vi "Test SendLogRecordsMakesThemAvailableInLoki.vi"(8 "error in (no error)":errorcluster) -> (0 "error out":errorcluster)   [LabVIEW 2017, in "UT_LokiHandler.lvlib"]
doc: "Template for an unit test with caraya in the \"Given, When, Then\" structure from James."
uses:
  UT_LokiHandler.lvlib
  Source/HSE-Logger/LogRecord/LogRecord.lvclass/LogRecord.ctl
  <vilib>/ErrorRing/Error Ring.xnode
  Source/HSE-Logger/Handler/LokiHandler/LokiHandler.lvclass
  <vilib>/addons/_JKI Toolkits/Caraya/classes/Test/Test.lvclass
  <vilib>/addons/_JKI Toolkits/Caraya/classes/Assert/Assert.lvclass
  Source/HSE-Logger/LogRecord/LogRecord.lvclass
  Source/HSE-Logger/LogLevel.ctl
  Source/HSE-Logger/hse-logger.lvlib
  <vilib>/Utility/error.llb/Error Cluster From Error Code.vi
  Source/HSE-Logger/Formatter/LokiJsonFormatter/LokiJsonFormatter.lvclass
  <vilib>/httpClient/LabVIEWHTTPClient.lvlib
  <vilib>/addons/_JKI Toolkits/Caraya/classes/Assert/Assert Greater_Variant.vi
  <vilib>/httpClient/POSTBuffer.vi
panel:
  # "Connector Pane"
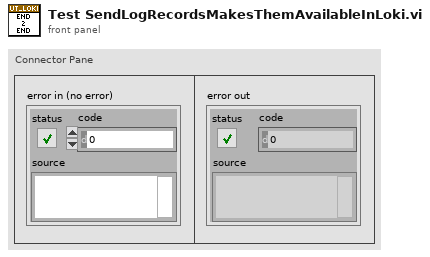
[diagram p1: front panel]
types:
  T1 = typedef "hse-logger.lvlib/LogLevel.ctl" = enum16{"DEBUG", "INFO", "WARNING", "ERROR", "CRITICAL"}
  T2 = typedef "LabVIEWHTTPClient.lvlib/ClientHandle.ctl" = refnum<k1>
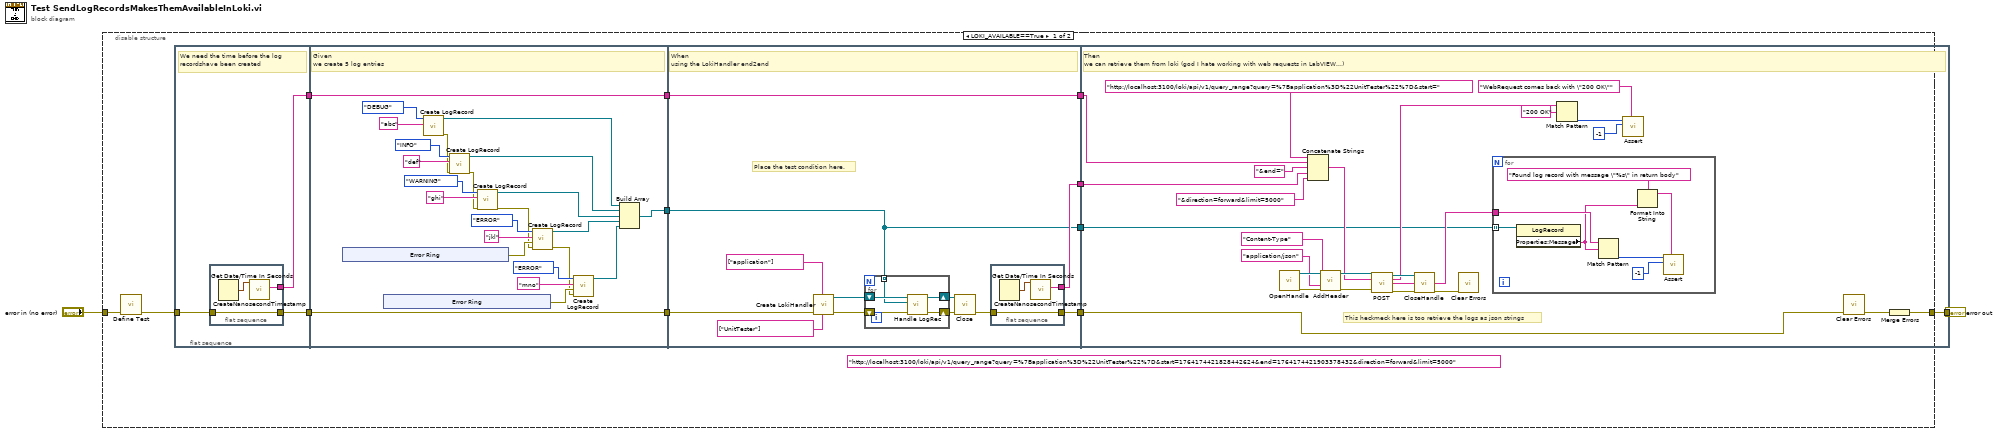
[diagram p0: block diagram]
diagram:
  n1 = disable-structure shown="LOKI_AVAILABLE==True" {
    disable-tunnel: [w12 w105] -> w2
    disable-tunnel: "error in (no error)" -> [w11 w105]
    frame condition #0 (active) {
      (unwired) "http://localhost:3100/loki/api/v1/query_range?query=%7Bapplication%3D%22UnitTester%22%7D&start=1764174421828442624&end=1764174421903378432&direction=forward&limit=5000" ("url")
      n2 = call <vilib>:"Define Test.vi"("error in (no error)"=w11) -> ("error out"=w10:errorcluster)  [unwired: 9 in, 1 out]
      n3 = flat-sequence {
        tunnel: w10 -> [w17]
        tunnel: [w16] -> w8
        tunnel: [w15] -> w5
        tunnel: [w44] -> w14
        tunnel: [w41] -> w9
        tunnel: w8 -> [w44]
        tunnel: [w22] -> w6
        tunnel: w5 -> [w22]
        tunnel: w14 -> [w56]
        tunnel: [w57] -> w13
        tunnel: w9 -> [w53]
        tunnel: [w55] -> w7
        tunnel: w6 -> [w55]
        tunnel: [w54] -> w4
        tunnel: [w53] -> w3
        tunnel: [w97] -> w12
        tunnel: w13 -> [w75]
        tunnel: w7 -> [w84]
        tunnel: w4 -> [w83]
        tunnel: w3 -> [w76]
        frame #0 {
          # "We need the time before the log recordshave been created"
          n4 = flat-sequence {
            tunnel: w17 -> [w20]
            tunnel: [w20] -> w16
            tunnel: [w18] -> w15
            frame #0 {
              n5 = Get Date/Time In Seconds() -> (seconds since 1Jan1904=w19:timestamp)
              n6 = call "CreateNanosecondTimestamp.vi"("current time"=w19) -> ("Timestring in RFC3339Nano"=w18:string)  [unwired: 9 in, 1 out]
            }
          }
        }
        frame #1 {
          # "Given\nwe create 5 log entries"
          n7 = xnode "Error Ring"() -> ("error out"=w31:errorcluster)
          n8 = xnode "Error Ring"() -> ("error out"=w30:errorcluster)
          n9 = call "Create LogRecord.vi"("Message"="abc", "Level"=LogLevel."DEBUG") -> ("error out"=w26:errorcluster, "LogRecord out"=w42:refnum<class "LogRecord.lvclass">)  [unwired: 8 in]
          n10 = call "Create LogRecord.vi"("error in"=w26, "Message"="def", "Level"=LogLevel."INFO") -> ("error out"=w25:errorcluster, "LogRecord out"=w38:refnum<class "LogRecord.lvclass">)  [unwired: 7 in]
          n11 = call "Create LogRecord.vi"("error in"=w25, "Message"="ghi", "Level"=LogLevel."WARNING") -> ("error out"=w24:errorcluster, "LogRecord out"=w35:refnum<class "LogRecord.lvclass">)  [unwired: 7 in]
          n12 = call "Create LogRecord.vi"("error in"=w24, "Error to Log"=w31, "Message"="jkl", "Level"=LogLevel."ERROR") -> ("error out"=w23:errorcluster, "LogRecord out"=w32:refnum<class "LogRecord.lvclass">)  [unwired: 6 in]
          n13 = call "Create LogRecord.vi"("error in"=w23, "Error to Log"=w30, "Message"="mno", "Level"=LogLevel."ERROR") -> ("LogRecord out"=w27:refnum<class "LogRecord.lvclass">)  [unwired: 6 in, 1 out]
          n14 = Build Array(w42, w38, w35, w32, w27) -> (w41:refnum<class "LogRecord.lvclass">[])
        }
        frame #2 {
          # "Place the test condition here."
          # "When\nusing the LokiHandler end2end"
          n15 = call "Create LokiHandler.vi"("Stream Fields Values"=string[] ["UnitTester"], "Stream Fields"=string[] ["application"], "error in"=w56) -> ("error out"=w62:errorcluster, "LokiHandler out"=w61:refnum<class "LokiHandler.lvclass">)  [unwired: 7 in]
          n16 = for {
            tunnel: w53 -> [w68] mode=indexing
            shift-right: [w70] -> w60
            shift-left: w62 -> [w72]
            shift-right: [w69] -> w59
            shift-left: w61 -> [w71]
            n17 = call-dynamic "Handle LogRec.vi"("error in"=w72, "LogRecord"=w68, "LokiHandler in"=w71) -> ("error out"=w70:errorcluster, "LokiHandler out"=w69:refnum<class "LokiHandler.lvclass">)  [unwired: 7 in]
          }
          n18 = call-dynamic "Close.vi"("error in"=w60, "LokiHandler in"=w59) -> ("error out"=w58:errorcluster)  [unwired: 8 in, 1 out]
          n19 = flat-sequence {
            tunnel: w58 -> [w67]
            tunnel: [w67] -> w57
            tunnel: [w65] -> w54
            frame #0 {
              n20 = Get Date/Time In Seconds() -> (seconds since 1Jan1904=w66:timestamp)
              n21 = call "CreateNanosecondTimestamp.vi"("current time"=w66) -> ("Timestring in RFC3339Nano"=w65:string)  [unwired: 9 in, 1 out]
            }
          }
        }
        frame #3 {
          # "This heckmeck here is too retrieve the logs as json strings"
          # "Then\nwe can retrieve them from loki (god I hate working with web requests in LabVIEW...)"
          n22 = call <vilib>:"OpenHandle.vi"() -> ("client handle out"=w93:T2, "error out"=w94:errorcluster)  [unwired: 14 in]
          n23 = Concatenate Strings("http://localhost:3100/loki/api/v1/query_range?query=%7Bapplication%3D%22UnitTester%22%7D&start=" ("url"), w84, "&end=" ("string"), w83, "&direction=forward&limit=5000") -> (w81:string)
          n24 = call <vilib>:"AddHeader.vi"("client handle"=w93, "header"="Content-Type", "value"="application/json", "error in (no error)"=w94) -> ("client handle out"=w90:T2, "error out"=w91:errorcluster)  [unwired: 10 in]
          n25 = call-poly <vilib>:"POST.vi"("client handle"=w90, "url"=w81, "error in (no error)"=w91) -> ("client handle out"=w89:T2, "headers"=w80:string, "body"=w77:string, "error out"=w88:errorcluster)  [unwired: 9 in]
          n26 = call <vilib>:"CloseHandle.vi"("client handle"=w89, "error in (no error)"=w88) -> ("error out"=w87:errorcluster)  [unwired: 13 in]
          n27 = call <vilib>:"Clear Errors.vi"("error in (no error)"=w87) -> ()  [unwired: 5 in, 2 out]
          n28 = for {
            tunnel: w77 -> [w99]
            tunnel: w76 -> [w104] mode=indexing
            n29 = property class="LogRecord"(reference=w104) -> ("Properties:Message"=w98:string)  [unwired: 1 in, 2 out]
            n30 = Match Pattern(string=w99, regular expression=w98) -> (offset past match=w101:i32)  [unwired: 1 in, 3 out]
            n31 = Format Into String(format string="Found log record with message \"%s\" in return body", w98) -> (resulting string=w102:string)  [unwired: 2 in, 1 out]
            n32 = call-poly <vilib>:"Assert.vi"("Label"=w102, "Actual"=-1 ("offset past match"), "Expected"=w101) -> ()  [unwired: 7 in, 2 out]
          }
          n33 = Match Pattern(string=w80, regular expression="200 OK") -> (offset past match=w74:i32)  [unwired: 1 in, 3 out]
          n34 = call-poly <vilib>:"Assert.vi"("Label"="WebRequest comes back with \"200 OK\"", "Actual"=-1 ("offset past match"), "Expected"=w74) -> ()  [unwired: 7 in, 2 out]
          n35 = call <vilib>:"Clear Errors.vi"("error in (no error)"=w75) -> ("error out"=w96:errorcluster)  [unwired: 5 in, 1 out]
          n36 = Merge Errors(w96) -> (w97:errorcluster)
        }
      }
    }
    frame condition #1 {
    }
  }
  "error out" <- w2
